vi "Send Termiation Notification on Error.vi"(8 "error in (no error)":errorcluster) -> (0 "error out":errorcluster)   [LabVIEW 2017]
doc: "On Error, send a termination notification."
uses:
  Utilities/Application Globals.vi
  <vilib>/Utility/SystemLogging/NI_SystemLogging.lvlib
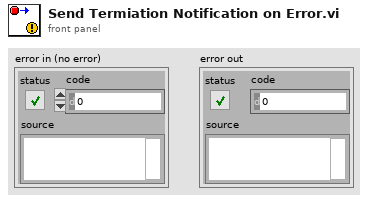
[diagram p1: front panel]
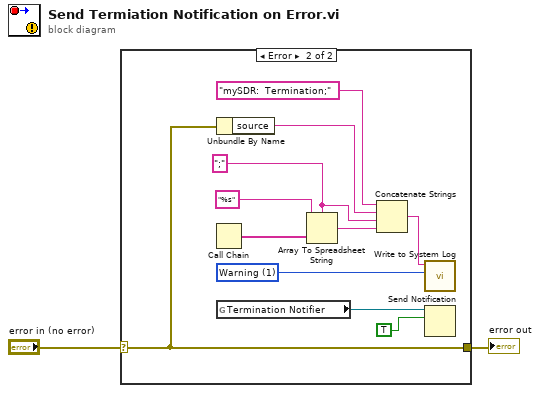
[diagram p0: block diagram]
diagram:
  n1 = case shown="Error" "error in (no error)" {
    selector: "error in (no error)" -> [w3 w7]
    tunnel: [w3 w7] -> w2
    frame No Error {
    }
    frame Error {
      w4 = ";" ("delimiter (Tab)")
      w12 = 1 items=["Error", "Warning", "Informational"] ("severity")
      n2 = Call Chain() -> (call chain=w11:string[])
      n3 = Unbundle By Name(w7) -> ("source"=w5:string)
      n4 = global read "Application Globals.vi" "Termination Notifier"() -> (w14:refnum<notifier>)
      n5 = Array To Spreadsheet String(delimiter (Tab)=w4, array=w11, 3:"%s" ("format string")) -> (spreadsheet string=w9:string)
      n6 = Concatenate Strings("mySDR:  Termination;", w5, w4, w9) -> (w8:string)
      n7 = call <vilib>:"Write to System Log.vi"("severity"=w12, "message"=w8) -> ()  [unwired: 9 in, 1 out]
      n8 = Send Notification(notification=TRUE, notifier=w14) -> ()  [unwired: 1 in, 2 out]
    }
  }
  "error out" <- w2
